vi "Search 1D Array for Nearest.vi"(9 "start index (0)":i32, 10 "desired element":dbl, 11 "1D Array":dbl[](array[numeric])) -> (1 "closest index":i32, 3 "closest element":dbl)   [LabVIEW 2014]
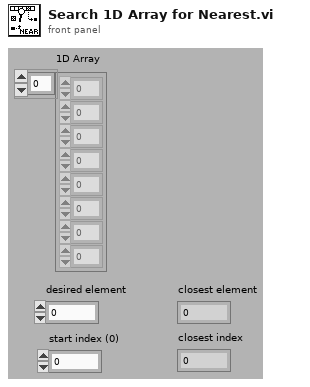
[diagram p1: front panel]
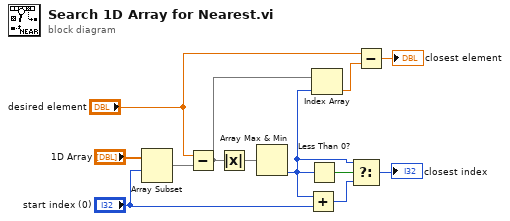
[diagram p0: block diagram]
diagram:
  n1 = Array Subset(array="1D Array", index="start index (0)") -> (w6:dbl[])  [unwired: 1 in]
  n2 = Subtract(x="desired element", y=w6) -> (x-y=w3:dbl[])
  n3 = Absolute Value(x=w3) -> (abs(x)=w10:dbl[])
  n4 = Array Max & Min(array=w10) -> (min index (indices)=w2:i32)  [unwired: 3 out]
  n5 = Add(x=w2, y="start index (0)") -> (x+y=w8:i32)
  n6 = Less Than 0?(x=w2) -> (x < 0?=w9:bool)
  n7 = Index Array(array=w3, index=w2) -> (element=w1:dbl)
  n8 = Select(t=w2, s=w9, f=w8) -> (s? t:f=→"closest index":i32)
  n9 = Subtract(x="desired element", y=w1) -> (x-y=→"closest element":dbl)
